vi "FPGA Messenger.vi"(6 "Sequence":fxp<+,16,16>, 7 "FPGA Action":T1, 8 "Duration":u32, 9 "Laser Mode":u16(ring) items=["Off", "On", "Rising", "Falling", "Camera"], 10 "Laser Channel":u16, 11 "Notifier Name":string) -> (0 "Duration":u32, 1 "Laser Mode":u16, 2 "Laser Channel":u16, 3 "Notifier Name Out":string, 4 "Sequence":fxp<+,16,16>, 5 "Write Confirm":bool)   [LabVIEW 2020]
uses:
  FPGA Controls/FPGA Action.ctl
  FPGA Controls/FPGA Notifier Element.ctl
  FPGA Controls/FPGA Laser Mode.ctl
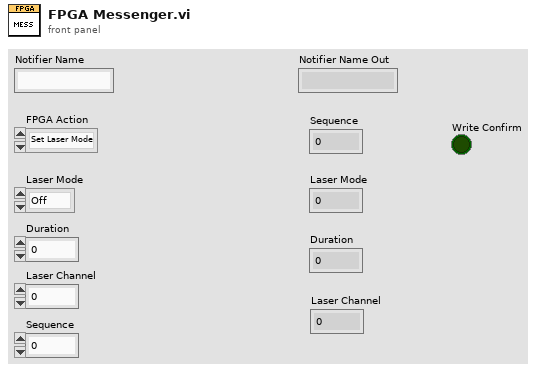
[diagram p1: front panel]
types:
  T1 = typedef "FPGA Action.ctl" = enum16{"Set Laser Mode", "Set Sequence", "Set Duration", "Write Check", "Idle", "Quit"}
  T2 = typedef "FPGA Notifier Element.ctl" = cluster{"Sequence":bool[], "Laser Mode":T3, "Duration":u32, "Laser Channel":u16, "Write Confirm ":bool, "Received?":bool, "FPGA Action":T1}
  T3 = typedef "FPGA Laser Mode.ctl" = u16
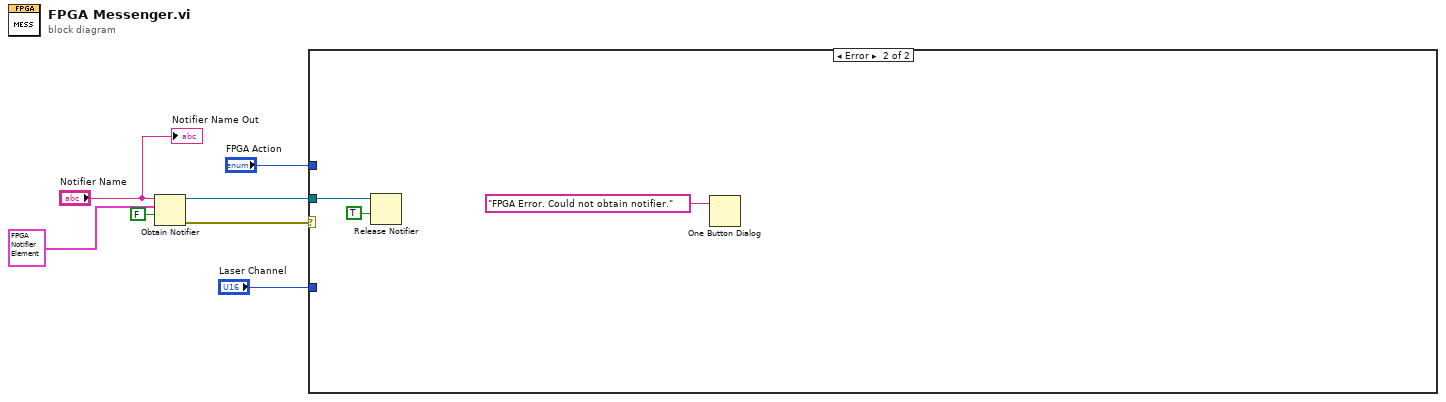
[diagram p0: block diagram]
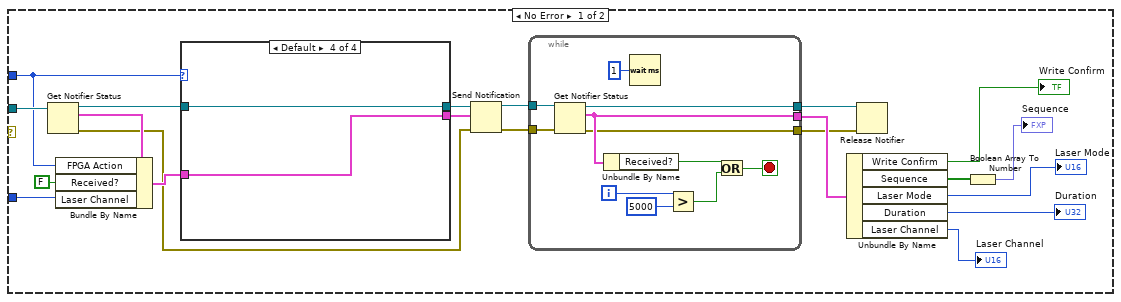
[diagram p2: hidden frame]
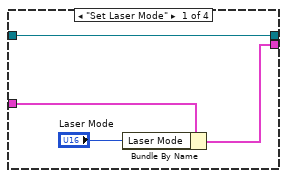
[diagram p3: hidden frame]
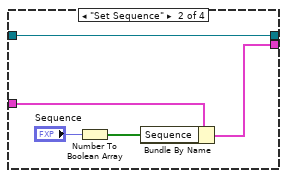
[diagram p4: hidden frame]
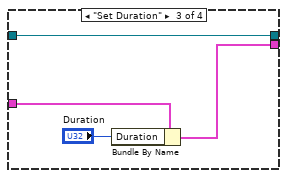
[diagram p5: hidden frame]
diagram:
  n1 = Obtain Notifier(name (unnamed)="Notifier Name", notification data type=T2 {"Sequence"=[], "Laser Mode"=0, "Duration"=0, "Laser Channel"=0, "Write Confirm "=FALSE, "Received?"=FALSE, "FPGA Action"=enum."Set Laser Mode"} ("Mojo Notifier Element"), create if not found? (T)=FALSE) -> (notifier out=w5:refnum<notifier>, error out=w6:errorcluster)  [unwired: 1 in, 1 out]
  n2 = case shown="Error" w6 {
    tunnel: w5 -> [w28 w56]
    tunnel: "FPGA Action" -> [w9 _]
    tunnel: "Laser Channel" -> [w8 _]
    frame No Error {
      n3 = Get Notifier Status(notifier=w28) -> (notifier out=w24:refnum<notifier>, current notification=w27:T2, error out=w18:errorcluster)  [unwired: 1 in, 2 out]
      n4 = Bundle By Name(cluster=w27, "FPGA Action"=w9, "Received?"=FALSE, "Laser Channel"=w8) -> (w25:T2)
      n5 = case shown="Default" w9 {
        tunnel: w25 -> [w43 w48 w52 w53]
        tunnel: [w41 w44 w49 w54] -> w23
        tunnel: w24 -> [w41 w44 w49 w54]
        tunnel: [w40 w45 w50 w53] -> w22
        frame "Set Laser Mode" {
          n6 = Bundle By Name(cluster=w43, "Laser Mode"="Laser Mode") -> (w40:T2)
        }
        frame "Set Sequence" {
          n7 = Number To Boolean Array(number="Sequence") -> (Boolean array=w47:bool[])
          n8 = Bundle By Name(cluster=w48, "Sequence"=w47) -> (w45:T2)
        }
        frame "Set Duration" {
          n9 = Bundle By Name(cluster=w52, "Duration"="Duration") -> (w50:T2)
        }
        frame Default {
        }
      }
      n10 = Send Notification(notification=w22, notifier=w23, error in (no error)=w18) -> (notifier out=w21:refnum<notifier>, error out=w17:errorcluster)
      n11 = while {
        tunnel: w21 -> [w38]
        tunnel: [w37] -> w19
        tunnel: [w31] -> w20
        tunnel: w17 -> [w30]
        tunnel: [w29] -> w16
        i -> [w35]
        stop <- w33 stop-if-true
        n12 = Get Notifier Status(notifier=w38, error in (no error)=w30) -> (notifier out=w37:refnum<notifier>, current notification=w31:T2, error out=w29:errorcluster)  [unwired: 2 out]
        n13 = Unbundle By Name(w31) -> ("Received?"=w36:bool)
        n14 = Wait (ms)(milliseconds to wait=u32 1) -> ()  [unwired: 1 out]
        n15 = Greater?(x=w35, y=5000) -> (0:w32:bool)
        n16 = Or(x=w36, y=w32) -> (x .or. y?=w33:bool)
      }
      n17 = Unbundle By Name(w20) -> ("Write Confirm"=→"Write Confirm":bool, "Sequence"=w15:bool[], "Laser Mode"=→"Laser Mode":T3, "Duration"=→"Duration":u32, "Laser Channel"=→"Laser Channel":u16)
      n18 = Release Notifier(notifier=w19, error in (no error)=w16) -> ()  [unwired: 1 in, 3 out]
      n19 = Boolean Array To Number(Boolean array=w15) -> (number=→"Sequence":fxp<+,16,16>)
    }
    frame Error {
      n20 = Release Notifier(notifier=w56, force destroy? (F)=TRUE) -> ()  [unwired: 1 in, 3 out]
      n21 = One Button Dialog(message="FPGA Error. Could not obtain notifier.") -> ()  [unwired: 1 in, 1 out]
    }
  }
  "Notifier Name Out" <- "Notifier Name"
